vi "WPI_CameraGetUSBImage.vi"(8 "error in (no error)":errorcluster, 10 "Refnum in":T1, 11 "Camera Address":string) -> (0 "error out":errorcluster, 2 "Refnum out":T1)   [LabVIEW 2017]
uses:
  <vilib>/vision/Image Controls.llb/IMAQ Image.ctl
  <vilib>/vision/driver/NI_Vision_Acquisition_Software.lvlib
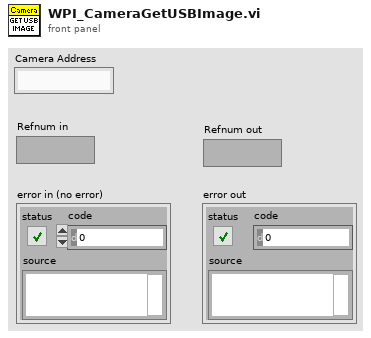
[diagram p1: front panel]
types:
  T1 = typedef "IMAQ Image.ctl" = refnum<image>
  T2 = typedef "IMAQdx.ctl" = refnum<k21>
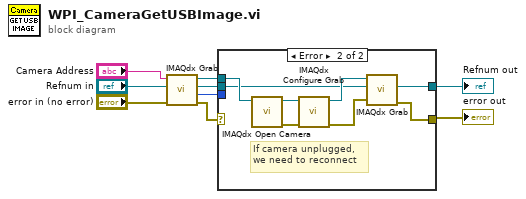
[diagram p0: block diagram]
diagram:
  n1 = call <vilib>:"IMAQdx Grab.vi"("error in"="error in (no error)", "Image In"="Refnum in", "Session In"="Camera Address") -> ("error out"=w4:errorcluster, "Buffer Number Out"=w2:u32, "Image Out"=w3:T1, "Session Out"=w1:T2)  [unwired: 5 in]
  n2 = case shown="Error" w4 {
    selector: w4 -> [w11 _]
    tunnel: [w11 w17] -> w8
    tunnel: w3 -> [w10 w12]
    tunnel: [w10 w13] -> w7
    tunnel: w2 -> [_ _]
    tunnel: w1 -> [_ w16]
    frame No Error {
    }
    frame Error {
      # "If camera unplugged,\nwe need to reconnect"
      n3 = call <vilib>:"IMAQdx Open Camera.vi"("Session In"=w16) -> ("error out"=w19:errorcluster, "Session Out"=w15:T2)  [unwired: 9 in]
      n4 = call <vilib>:"IMAQdx Configure Grab.vi"("error in"=w19, "Session In"=w15) -> ("error out"=w18:errorcluster, "Session Out"=w14:T2)  [unwired: 8 in]
      n5 = call <vilib>:"IMAQdx Grab.vi"("error in"=w18, "Image In"=w12, "Session In"=w14) -> ("error out"=w17:errorcluster, "Image Out"=w13:T1)  [unwired: 5 in, 2 out]
    }
  }
  "error out" <- w8
  "Refnum out" <- w7
